vi "poly_inv_solve.vi"(6 "Default":dbl, 8 "upper limit":dbl=1.0, 9 "lower limit":dbl=-1.0, 10 "y":dbl, 11 "P(x)":dbl[](array[numeric])) -> (2 "x":dbl, 3 "All x":dbl[](array[numeric]))   [LabVIEW 2013]
uses:
  <vilib>/Analysis/polynomials.llb/Polynomial Roots (DBL).vi
  <vilib>/Analysis/NI_AALPro.lvlib
panel:
  # "Number of times the x value is reached on the interval."
  # "All values at which P(x) = y."
  # "One x value, or Default if no solutions on the interval."
  # "Given polynomial and Y value, find corresponding X value on the specified interval.   Since a polynomial cannot in general be inverted, the specified value may not be reached on that interval, or there may be more than one crossing."
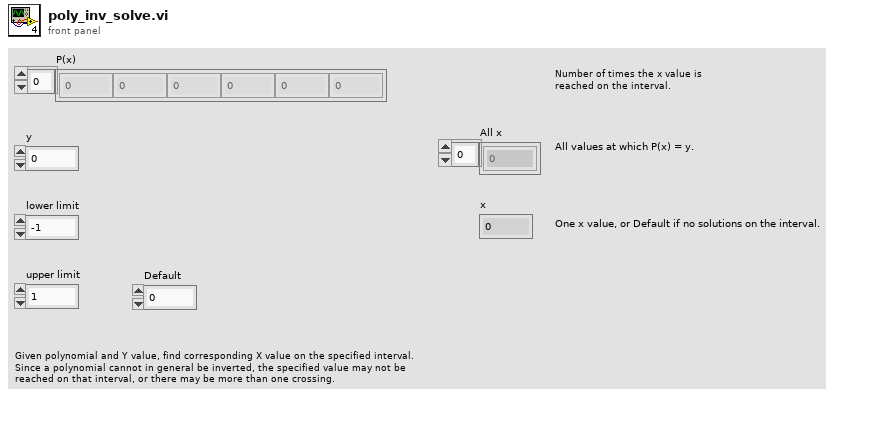
[diagram p1: front panel]
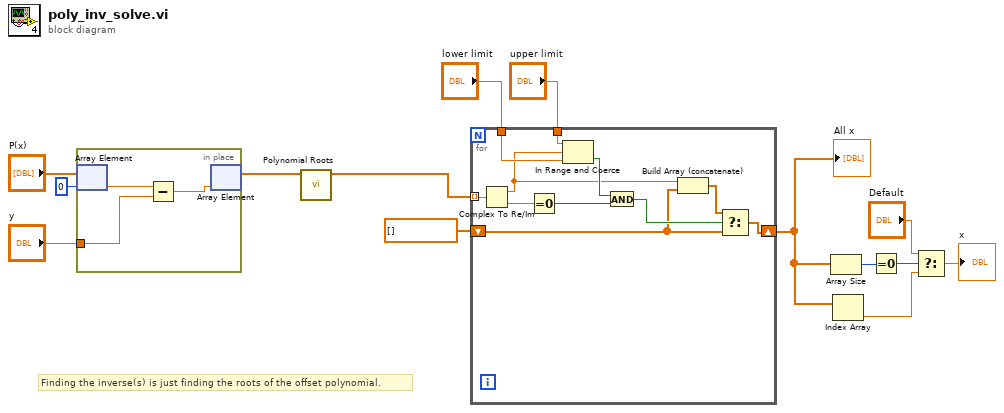
[diagram p0: block diagram]
diagram:
  # "Finding the inverse(s) is just finding the roots of the offset polynomial."
  n1 = in-place {
    in-place-border: "y" -> [w16]
    n2 = in-place-array #1("P(x)", 0) -> (w17:dbl)
    n3 = Subtract(x=w17, y=w16) -> (x-y=w15:dbl)
    n4 = in-place-array #1(w15) -> (w11:dbl[])  [unwired: 1 out]
  }
  n5 = call-poly <vilib>:"Polynomial Roots.vi"("P(x)"=w11) -> ("Roots"=w14:cdb[])  [unwired: 9 in, 1 out]
  n6 = for {
    tunnel: w14 -> [w28] mode=indexing
    shift-right: [w18] -> w2
    shift-left: dbl[] [] ("Roots") -> [w20]
    tunnel: "upper limit" -> [w24]
    tunnel: "lower limit" -> [w23]
    n7 = Complex To Re/Im(x + iy=w28) -> (x=w21:dbl, y=w27:dbl)
    n8 = Equal To 0?(x=w27) -> (x = 0?=w25:bool)
    n9 = In Range and Coerce(upper limit=w24, x=w21, lower limit=w23) -> (In Range?=w26:bool)  [unwired: 1 out]
    n10 = And(x=w26, y=w25) -> (x .and. y?=w22:bool)
    n11 = Build Array (concatenate)(w21, w20) -> (w19:dbl[])
    n12 = Select(t=w19, s=w22, f=w20) -> (s? t:f=w18:dbl[])
  }
  "All x" <- w2
  n13 = Array Size(array=w2) -> (size(s)=w6:i32)
  n14 = Index Array(array=w2) -> (element=w1:dbl)  [unwired: 1 in]
  n15 = Equal To 0?(x=w6) -> (x = 0?=w4:bool)
  n16 = Select(t="Default", s=w4, f=w1) -> (s? t:f=→"x":dbl)
